vi "Default Log File--constant.vi"() -> (3 "Default Log File":path)   [LabVIEW 2025]
doc: "This constant defines the default log file for the export strings method."
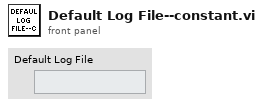
[diagram p1: front panel]
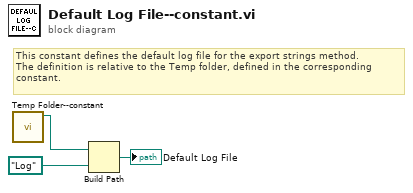
[diagram p0: block diagram]
diagram:
  # "This constant defines the default log file for the export strings method.\nThe definition is relative to the Temp folder, defined in the corresponding\nconstant."
  n1 = call "Temp Folder--constant.vi"() -> ("Temp Folder"=w1:path)  [unwired: 7 in]
  n2 = Build Path(base path=w1, name or relative path=path "Log" ("Test Folder")) -> (appended path=→"Default Log File":path)
